vi "myRIO_BRig_RT_dataExp_Tcycle_RewardPost.vi"() -> (2 "output_Tcycle_RewardPost":i32)   [LabVIEW 2014]
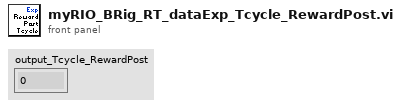
[diagram p1: front panel]
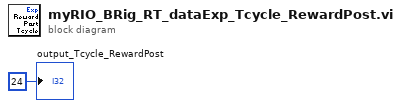
[diagram p0: block diagram]
diagram:
  "output_Tcycle_RewardPost" <- 24 ("output_iBlock")
